vi "get desired labview version.vi"(11 "command line arguments":T1) -> (3 "lv version":dbl)   [LabVIEW 2013]
uses:
  arguments.ctl
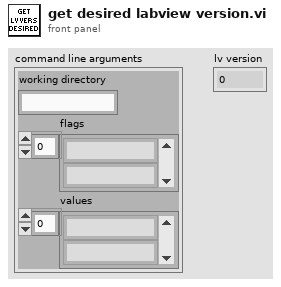
[diagram p1: front panel]
types:
  T1 = typedef "arguments.ctl" = cluster{"working directory":string, "flags":string[], "values":string[]}
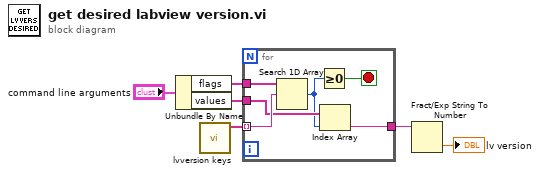
[diagram p0: block diagram]
diagram:
  n1 = Unbundle By Name("command line arguments") -> ("flags"=w4:string[], "values"=w3:string[])
  n2 = call "lvversion keys.vi"() -> ("lv version keys"=w2:string[])  [unwired: 11 in]
  n3 = for {
    tunnel: w4 -> [w12]
    tunnel: w3 -> [w10]
    tunnel: w2 -> [w11] mode=indexing
    tunnel: [w9] -> w1
    stop <- w7 stop-if-true
    n4 = Search 1D Array(1D array=w12, element=w11) -> (index of element=w8:i32)  [unwired: 1 in]
    n5 = Greater Or Equal To 0?(x=w8) -> (x >= 0?=w7:bool)
    n6 = Index Array(array=w10, index=w8) -> (element=w9:string)
  }
  n7 = Fract/Exp String To Number(string=w1) -> (number=→"lv version":dbl)  [unwired: 3 in, 1 out]
